vi "1作业.vi"() -> ()   [LabVIEW 2018]
panel:
  in  "停止":bool
  out "文本显示":string="NIHAOA。\n大计、党之大计，是民族振兴、社会进步的重要基石。党的十八大以来，以习近平同志为核心的党中央高度重视教育事业，我国教育事业取得了历史性成就。如今，我国已建成世界最大规模且有质量的教育体系。这些成就让我深刻认识到，教育强国建设是实现中华民族伟大复兴的基础工程。作为新时代的大学生党员，我们要充分认识教育强国的重要意义，珍惜来之不易的教育机会，努力学习科学文化知识，不断提升自身综合素质，为实现教育强国梦贡献自己的力量。2333的力量。"
  in  "操作(0:open)":T1(ring)=enum."open or create"
  in  "文件路径（使用对话框）":path=path "D:/Desktop/work/虚拟仪器技术/class/3.24/作业/3.24zuoye.txt"
  in  "文本输入":string="NIHAOA。"
  in  "字幕内容":string="加油好男儿"
  out "?":bool[][](array[boolean])
  in  "滚动速度":u32=10
  in  "滚动方式":enum32{"左", "暂停", "右"}(radio)
  in  "停止按钮":bool
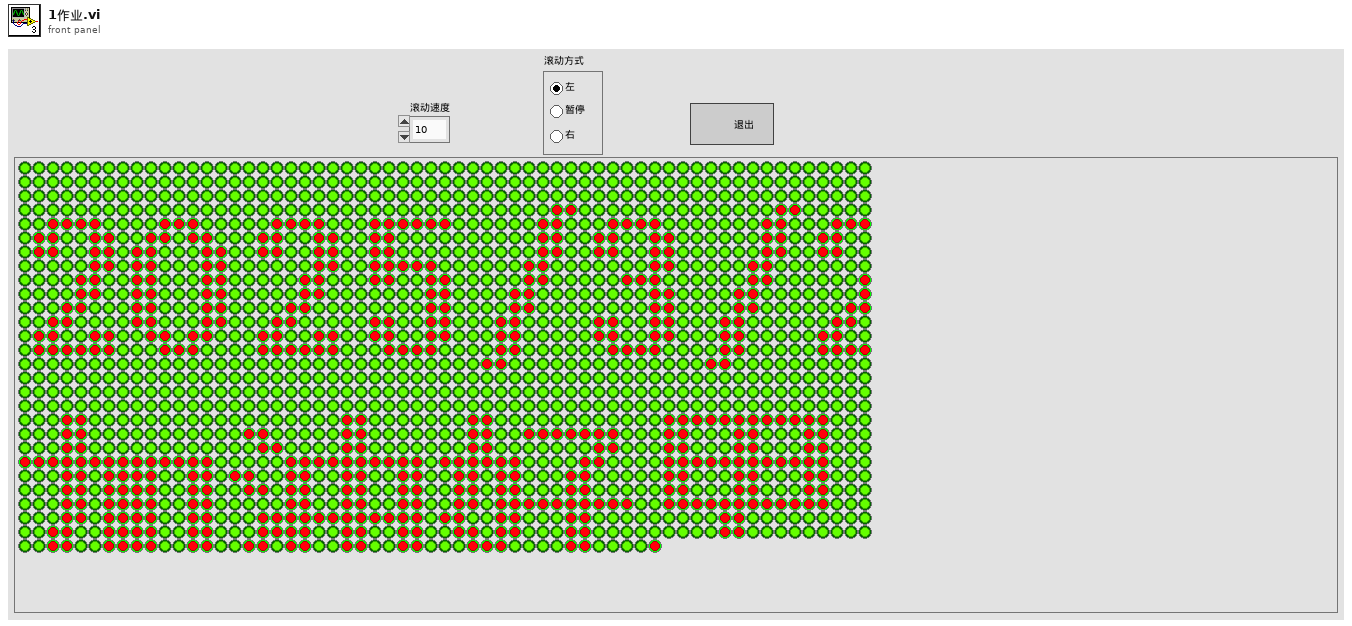
[diagram p1: front panel]
types:
  T1 = enum16{"open", "replace", "create", "open or create", "replace or create", "replace or create with confirmation"}
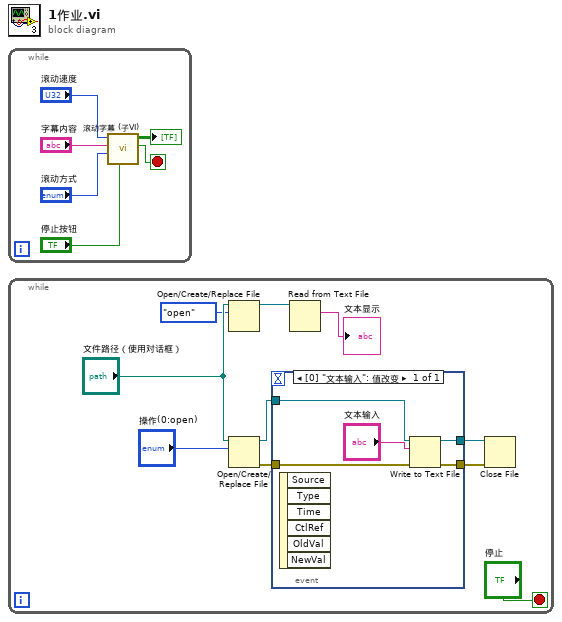
[diagram p0: block diagram]
diagram:
  n1 = while {
    stop <- w1 stop-if-true
    n2 = call "滚动字幕 (子VI).vi"("停止按钮输入"="停止按钮", "滚动方式"="滚动方式", "字幕内容"="字幕内容", "滚动速度"="滚动速度") -> ("停止按钮输出"=w1:bool, 3:→"?":bool[][])  [unwired: 6 in]
  }
  n3 = while {
    stop <- "停止" stop-if-true
    n4 = Open/Create/Replace File(file path (use dialog)="文件路径（使用对话框）", operation (0:open)=T1."open" ("操作(0:open) 2")) -> (refnum out=w8:refnum<file>)  [unwired: 4 in, 2 out]
    n5 = Open/Create/Replace File(file path (use dialog)="文件路径（使用对话框）", operation (0:open)="操作(0:open)") -> (refnum out=w10:refnum<file>, error out=w11:errorcluster)  [unwired: 4 in, 1 out]
    n6 = event shown="[0] \"文本输入\": 值改变" {
      selector: _ -> [_]
      dyn-events: _ -> [_]
      timeout: _ -> [_]
      tunnel: [w20] -> w14
      tunnel: [w19] -> w13
      tunnel: w11 -> [w18]
      tunnel: w10 -> [w17]
      event "文本输入": Value Change {
        n7 = event-data() -> ()  [unwired: 1 in, 6 out]
        n8 = Write to Text File(file (use dialog)=w17, text="文本输入", error in=w18) -> (refnum out=w19:refnum<file>, error out=w20:errorcluster)  [unwired: 1 in, 1 out]
      }
    }
    n9 = Read from Text File(file (use dialog)=w8) -> (text=→"文本显示":string)  [unwired: 3 in, 3 out]
    n10 = Close File(refnum=w13, error in=w14) -> ()  [unwired: 2 out]
  }
